vi "initialize Session Data.vi"(0 "OBJ - Session in":refnum<class "File Session.lvclass">=refnum, 11 "error in":errorcluster) -> (4 "OBJ - Session out":refnum<class "File Session.lvclass">, 15 "error out":errorcluster)   [LabVIEW 2016, in "File Session.lvclass"]
doc: "OVERRIDE VI\nPlaceholder for decendant sessions to initialize and set their default values"
uses:
  File Session.lvclass
  Accessors/Read Path.vi
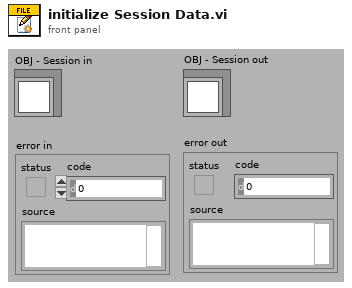
[diagram p1: front panel]
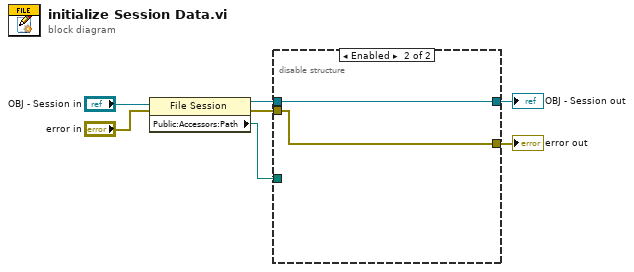
[diagram p0: block diagram]
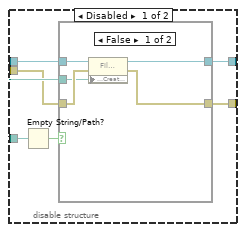
[diagram p2: hidden frame]
diagram:
  n1 = property class="File Session"(reference="OBJ - Session in", error in="error in") -> (reference out=w5:refnum<class "File Session.lvclass">, error out=w3:errorcluster, "Public:Accessors:Path"=w4:path)
  n2 = disable-structure shown="Enabled" {
    disable-tunnel: w5 -> [w12 w22]
    disable-tunnel: w4 -> [w11 _]
    disable-tunnel: w3 -> [w10 w21]
    disable-tunnel: [w9 w22] -> w2
    disable-tunnel: [w8 w21] -> w1
    frame Disabled {
      n3 = Empty String/Path?(string/path=w11) -> (empty?=w13:bool)
      n4 = case shown="False" w13 {
        tunnel: w11 -> [w14 _]
        tunnel: w10 -> [w18 w19]
        tunnel: w12 -> [w17 w20]
        tunnel: [w16 w20] -> w9
        tunnel: [w15 w19] -> w8
        frame False {
          n5 = property class="File Session"(reference=w17, error in=w18, "Public:Create (Replace) File"=w14) -> (reference out=w16:refnum<class "File Session.lvclass">, error out=w15:errorcluster)
        }
        frame True {
          # "If no file is present, don't try to open..."
        }
      }
    }
    frame Enabled {
    }
  }
  "error out" <- w1
  "OBJ - Session out" <- w2
